vi "Actor Core.vi"(8 "error in":errorcluster, 11 "Contestant in":refnum<class "Contestant.lvclass">) -> (0 "error out":errorcluster, 3 "Actor out":refnum<class "Actor.lvclass">)   [LabVIEW 2024, in "Contestant.lvlib" / "Contestant.lvclass"]
doc: "<p>(<strong>Filename</strong>: <span class=\"dnl\">Actor Framework.lvlib:Actor.lvclass:Actor Core.vi</span>)</p>\n<p>Receives messages to the actor, reacts to them, and initiates any error handling that may shut the actor down.</p>\n<p>Descendant classes may override this VI to append parallel tasks for the actor to complete while it handles messages. Overrides use the <a href=\"nihelplauncher://docs/csh?context=lvcore_glang_udclass\">Call Parent Class Method</a> node.</p>"
uses:
  Contestant.lvclass
  <vilib>/ActorFramework/Actor/Actor.lvclass
  Applications/National Instruments/LabVIEW 2024 64-bit/vi.lib/ActorFramework/Actor/Actor.lvclass
  Contestant.lvclass/Contestant.ctl
  <vilib>/ActorFramework/Actor/Actor.lvclass/Actor.ctl
  Controller/Controller Messages/Load Contestant Panel Msg/Load Contestant Panel Msg.lvclass/Load Contestant Panel Msg.ctl
  <vilib>/ActorFramework/Message Enqueuer/Message Enqueuer.lvclass/Message Enqueuer.ctl
  <vilib>/ActorFramework/Message Enqueuer/Enqueue.vi
  Controller/Controller Messages/Load Contestant Panel Msg/Load Contestant Panel Msg.lvclass
  Applications/National Instruments/LabVIEW 2024 64-bit/vi.lib/ActorFramework/Message/Message.lvclass
  <vilib>/ActorFramework/Message Priority Queue/Priority Enqueue.vi
panel:
  out "Contestant Name":string="NAME"
  out "Contestant Score":string="000"
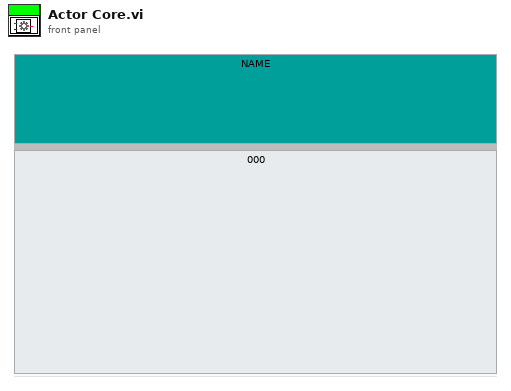
[diagram p1: front panel]
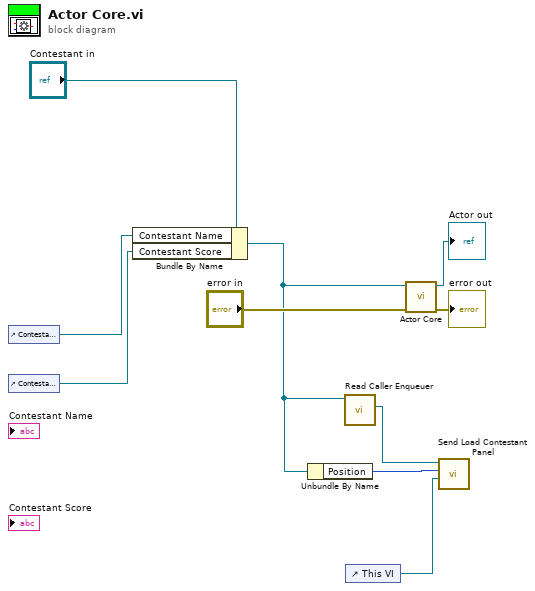
[diagram p0: block diagram]
diagram:
  n1 = control-ref of="Contestant Name"() -> (w6:refnum<vi>)
  n2 = control-ref of="Contestant Score"() -> (w5:refnum<vi>)
  n3 = Bundle By Name(cluster="Contestant in", "Contestant Name"=w6, "Contestant Score"=w5) -> (w2:refnum<class "Contestant.lvclass">)
  n4 = Unbundle By Name(w2) -> ("Position"=w1:i32)
  n5 = call <vilib>:"Read Caller Enqueuer.vi"("Actor"=w2) -> ("Caller Enqueuer"=w4:refnum<class "Message Enqueuer.lvclass">)  [unwired: 10 in]
  n6 = control-ref of="This VI"() -> (w3:refnum<vi>)
  n7 = call-parent "Actor Core.vi"("error in"="error in", "Actor in"=w2) -> ("error out"=→"error out":errorcluster, "Actor out"=→"Actor out":refnum<class "Actor.lvclass">)  [unwired: 8 in]
  n8 = call "Send Load Contestant Panel.vi"("VI Ref"=w3, "Contestant"=w1, "Message Enqueuer"=w4) -> ()  [unwired: 7 in, 2 out]
